vi "Write Data.vi"(8 "error in (no error)":errorcluster, 10 "Base Data Lib:Single_Array.lvclass":refnum<class "Single_Array.lvclass">, 11 "Update Humidifier Output Data MSG in":refnum<class "Update Humidifier Output Data MSG.lvclass">) -> (0 "error out":errorcluster, 3 "Update Humidifier Output Data MSG out":refnum<class "Update Humidifier Output Data MSG.lvclass">)   [LabVIEW 2014, in "Update Humidifier Output Data MSG.lvclass"]
uses:
  Update Humidifier Output Data MSG.lvclass
  reusable/Data/Array Data/Single 1-D/Single_Array.lvclass
  Update Humidifier Output Data MSG.lvclass/Update Humidifier Output Data MSG.ctl
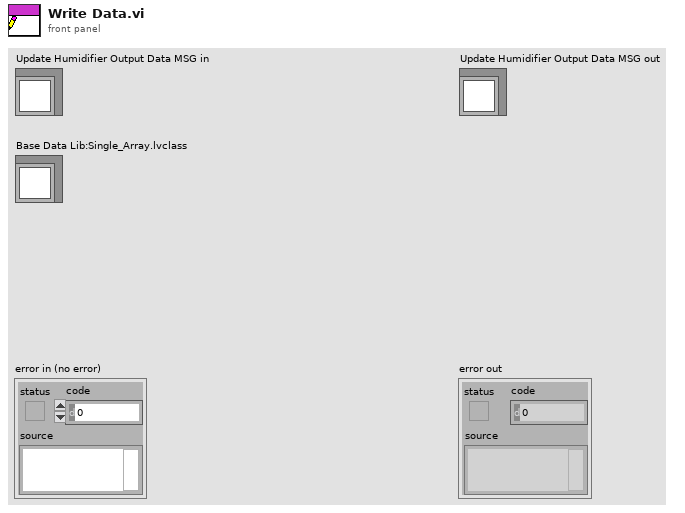
[diagram p1: front panel]
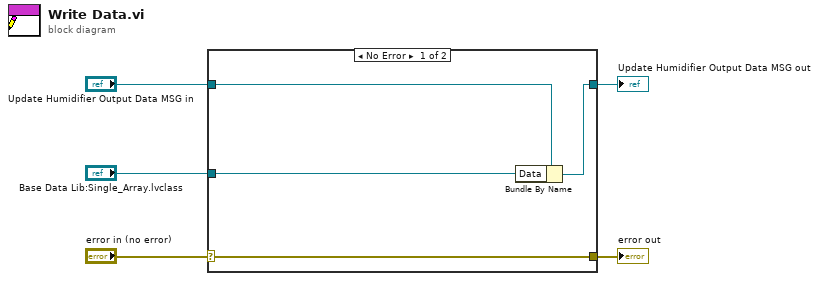
[diagram p0: block diagram]
diagram:
  n1 = case shown="No Error" "error in (no error)" {
    selector: "error in (no error)" -> [w9 w10]
    tunnel: [w9 w10] -> w4
    tunnel: [w7 w11] -> w2
    tunnel: "Update Humidifier Output Data MSG in" -> [w8 w11]
    tunnel: "Base Data Lib:Single_Array.lvclass" -> [w6 _]
    frame No Error {
      n2 = Bundle By Name(cluster=w8, "Data"=w6) -> (w7:refnum<class "Update Humidifier Output Data MSG.lvclass">)
    }
    frame Error {
    }
  }
  "error out" <- w4
  "Update Humidifier Output Data MSG out" <- w2
